vi "UHR-Fleezers Control (host) - 10.8.vi"() -> ()   [LabVIEW 2013] (continued)
            n1214 = xnode "Read/Write Control"("FPGA VI Reference In"=w3569, "error in"=w3568, "AI to FIFO"=w3570, "APD to FIFO"=w3570, "Start scan"=w3570) -> ("FPGA VI Reference Out"=w3567:T19, "error out"=w3566:errorcluster)
          }
          frame True {
            w3594 = FALSE ("1D or 2D Scan?")
            w3599 = TRUE ("AI to FIFO")
            # "Count for MCL loop"
            # "N total cycles"
            # "N steps"
            # "V_int"
            n1215 = local read "Scan Range (nm)"() -> (w3576:dbl)
            n1216 = local read "Number of F/B Scans (AOD)"() -> (w3593:u16)
            n1217 = Sign(1:w3576) -> (0:w3575:dbl)
            n1218 = Compound Arithmetic op=MULTIPLY(w3576, "MCL Step Position Ratio", "MCL/AOM Scale Tweak") -> (w3580:dbl)
            n1219 = Negate(x=w3575) -> (-x=w3572:dbl)
            n1220 = Multiply(x=w3572, y="MCL Step Increment (V_int)") -> (x*y=w3574:dbl)
            n1221 = Divide(x=w3580, y="MCL X Cal (nm/V)") -> (x/y=w3586:dbl)
            n1222 = Multiply(x=32767.0 ("y"), y=w3586) -> (x*y=w3592:dbl)
            n1223 = local read "Total Counts (ticks)"() -> (w3577:u32)
            n1224 = local read "Cycles/step (AOD)"() -> (w3588:u64)
            n1225 = local read "Scan steps (AOD)"() -> (w3589:u64)
            n1226 = Divide(x=w3592, y=10.0) -> (x/y=w3585:dbl)
            n1227 = Divide(x=w3585, y="MCL Step Increment (V_int)") -> (x/y=w3583:dbl)
            n1228 = Absolute Value(x=w3583) -> (abs(x)=w3571:dbl)
            n1229 = Compound Arithmetic op=MULTIPLY(w3589, w3588, w3577) -> (w3584:u64)
            n1230 = local write "wait to reset values"(w3599) -> ()
            n1231 = local write "MCL Scanning"(w3599) -> ()
            n1232 = Divide(x=w3584, y=w3571) -> (x/y=w3581:dbl)
            "MCL Count" <- w3581
            n1233 = xnode "Read/Write Control"("FPGA VI Reference In"=w3598, "error in"=w3597, "Scan steps (MCL)"=w3571, "Number of scans (MCL)"=w3593, "Cycles per step (MCL)"=u64 1, "Scan freq.  increment (MCL)"=w3574, "1D or 2D Scan?"=w3594, "MCL Scan Axis"=w3594, "Cont. Scan (MCL)"=w3594, "MCL count"=w3581) -> ("FPGA VI Reference Out"=w3596:T19, "error out"=w3595:errorcluster)
            n1234 = xnode "Read/Write Control"("FPGA VI Reference In"=w3596, "error in"=w3595, "AI to FIFO"=w3599, "APD to FIFO"=w3599, "Start scan"=w3599, "Start scan (MCL)"=w3599) -> ("FPGA VI Reference Out"=w3601:T19, "error out"=w3600:errorcluster)
          }
        }
        "Raster Scanning..." <- TRUE ("Scanning...")
      }
    }
    n1235 = And(x="Save scans", y=w2105) -> (x .and. y?=w2151:bool)
    n1236 = Compound Arithmetic op=OR("Start MCL Scan", "Confocal Image", "Confocal Linescan") -> (w2103:bool)
    n1237 = And(x="Save Data (MCL)", y=w2103) -> (x .and. y?=w2150:bool)
    n1238 = case "Start MCL raster scan" shown="True" w2103 {
      tunnel: w2153 -> [w3032 w3047]
      tunnel: w2152 -> [w3031 w3046]
      tunnel: [w3032 w3042] -> w1910
      tunnel: [w3031 w3041] -> w1909
      tunnel: [FALSE w3040] -> w2136
      tunnel: "Start MCL Scan" -> [_ w3035]
      tunnel: "Confocal Image" -> [_ w3034]
      tunnel: "Confocal Linescan" -> [_ _]
      frame False {
      }
      frame True {
        w3040 = TRUE
        n1239 = case shown="True" "Restart DMA? (MCL)" {
          tunnel: [w3092 w3094] -> w3045
          tunnel: [w3091 w3093] -> w3044
          tunnel: w3047 -> [w3092 w3097]
          tunnel: w3046 -> [w3091 w3096]
          frame False {
          }
          frame True {
            n1240 = call "reset FPGA DMA.vi"("error in"=w3096, "FPGA VI Reference In"=w3097) -> ("error out"=w3093:errorcluster, "FPGA VI Reference Out"=w3094:T19)
            n1241 = local write "Overflow (data lost)"(FALSE ("Overflow (data lost)")) -> ()
          }
        }
        n1242 = case shown="False" w3035 {
          selector: w3035 -> [_ w3051]
          tunnel: w3034 -> [w3050 _]
          tunnel: [w3050 w3051] -> w3033
          frame False {
            n1243 = property on="2D or 1D Scan" class="Bool (strict)"("Val(Sgnl)"=w3050) -> ()  [unwired: 2 in, 2 out]
            n1244 = property on="Confocal Image" class="Bool (strict)"("Value"=FALSE ("Start Confocal Map")) -> ()  [unwired: 2 in, 2 out]
          }
          frame True {
          }
        }
        n1245 = local write "MCL Scanning"(w3040) -> ()
        n1246 = local read "AO1"() -> (w3037:dbl)
        n1247 = local read "AO2"() -> (w3036:dbl)
        n1248 = case shown="True" "Center Scan" {
          tunnel: w3045 -> [w3058 w3090]
          tunnel: w3044 -> [w3057 w3089]
          tunnel: [w3056 w3088] -> w3042
          tunnel: [w3055 w3087] -> w3041
          tunnel: [w3053 w3074] -> w3039
          tunnel: [w3052 w3073] -> w3038
          tunnel: w3037 -> [w3053 w3079]
          tunnel: w3036 -> [w3052 w3082]
          tunnel: w3033 -> [_ _]
          frame False {
            w3054 = TRUE ("AI to FIFO")
            n1249 = xnode "Read/Write Control"("FPGA VI Reference In"=w3058, "error in"=w3057, "AI to FIFO"=w3054, "APD to FIFO"=w3054, "Start scan (MCL)"=w3054) -> ("FPGA VI Reference Out"=w3056:T19, "error out"=w3055:errorcluster)
          }
          frame True {
            w3086 = TRUE ("AI to FIFO")
            n1250 = local read "Scan steps (MCL)"() -> (w3065:u64)
            n1251 = local read "Scan lines (y)"() -> (w3061:u64)
            n1252 = local read "Fast Scan Dir"() -> (w3072:bool)
            n1253 = local read "Actual MCL Inc (V)"() -> (w3062:dbl)
            n1254 = Decrement(x=w3061) -> (x-1=w3060:u64)
            n1255 = Decrement(x=w3065) -> (x-1=w3064:u64)
            n1256 = Multiply(x=w3062, y=w3060) -> (x*y=w3059:dbl)
            n1257 = Divide(x=w3059, y=2.0) -> (x/y=w3069:dbl)
            n1258 = Multiply(x=w3062, y=w3064) -> (x*y=w3063:dbl)
            n1259 = Divide(x=w3063, y=2.0) -> (x/y=w3068:dbl)
            n1260 = Select(t=w3068, s=w3072, f=w3069) -> (s? t:f=w3067:dbl)
            n1261 = Select(t=w3069, s=w3072, f=w3068) -> (s? t:f=w3071:dbl)
            n1262 = Subtract(x=w3079, y=w3071) -> (x-y=w3070:dbl)
            n1263 = Subtract(x=w3082, y=w3067) -> (x-y=w3066:dbl)
            n1264 = local read "2D or 1D Scan"() -> (w3084:bool)
            n1265 = Not(x=w3072) -> (.not. x?=w3078:bool)
            n1266 = Not(x=w3084) -> (.not. x?=w3080:bool)
            n1267 = And(x=w3072, y=w3080) -> (x .and. y?=w3081:bool)
            n1268 = And(x=w3080, y=w3078) -> (x .and. y?=w3083:bool)
            n1269 = Select(t=w3082, s=w3083, f=w3066) -> (s? t:f=w3073:dbl)
            n1270 = Select(t=w3079, s=w3081, f=w3070) -> (s? t:f=w3074:dbl)
            n1271 = call "Volt to I16.vi"("Voltage In"=w3074) -> ("I16 Voltage Out"=w3077:i16)
            n1272 = call "Volt to I16.vi"("Voltage In"=w3073) -> ("I16 Voltage Out"=w3076:i16)
            n1273 = xnode "Read/Write Control"("FPGA VI Reference In"=w3090, "error in"=w3089, "AI to FIFO"=w3086, "APD to FIFO"=w3086, "Start scan (MCL)"=w3086, "AO1"=w3077, "AO2"=w3076) -> ("FPGA VI Reference Out"=w3088:T19, "error out"=w3087:errorcluster)
          }
        }
        "Initial Y" <- w3039
        "Initial X" <- w3038
        "wait to reset values" <- w3040
      }
    }
    n1274 = local read "Trap Pos Elements/DMA read"() -> (w1984:u32)
    n1275 = local read "Trap AI Elements/DMA read"() -> (w1908:u32)
    n1276 = local read "APD Elements/DMA read"() -> (w2027:u32)
    n1277 = local read "Trap AI FIFO Depth"() -> (w2200:u32)
    n1278 = xnode "Invoke Method"("FPGA VI Reference In"=w1910, "error in"=w1909, "Number of Elements"=w1984, "Timeout (ms)"=-1) -> ("Data"=w1948:u16[], "Elements Remaining"=→"Trap Pos FIFO El Remaining":u32)  [unwired: 2 out]
    n1279 = xnode "Invoke Method"("FPGA VI Reference In"=w1910, "error in"=w1909, "Number of Elements"=w1908, "Timeout (ms)"=-1 ("Timeout")) -> ("FPGA VI Reference Out"=w1912:T19, "error out"=w1911:errorcluster, "Data"=w1907:i16[], "Elements Remaining"=w1913:u32)
    "Trap AI FIFO El. Rem." <- w1913
    n1280 = xnode "Get APD Data"("FPGA VI Reference In"=w1910, "error in"=w1909, "Number of Elements"=w2027, "Timeout (ms)"=-1) -> ("Data"=w2026:u32[], "Elements Remaining"=→"APD FIFO Elements Remaining":u32)  [unwired: 2 out]
    n1281 = Subtract(x=w2200, y=w1908) -> (x-y=w2199:u32)
    n1282 = Decimate 1D Array(w1948) -> (w1945:u16[], w1947:u16[], w1946:u16[])
    n1283 = Divide(x=w1913, y=w2199) -> (x/y=w2198:dbl)
    "Buffer Status" <- w2198
    n1284 = To Unsigned Long Integer(number=w1945) -> (unsigned 32bit integer=w1944:u32[])
    n1285 = Join Numbers(hi=w1947, lo=w1946) -> ((hi.lo)=w1943:u32[])
    n1286 = Equal?(x=w2198, y=1.0) -> (x = y?=w2196:bool)
    n1287 = Join Numbers(hi=w1944, lo=w1943) -> ((hi.lo)=w1937:u64[])
    n1288 = call "IR AOM word to freq - vec.vi"("Frequency Word In (double vec)"=w1937) -> ("Frequency Out"=w1983:dbl[])
    n1289 = case "Alert buffer overflow" shown="True" w2196 {
      frame False {
      }
      frame True {
        n1290 = call <vilib>:"Beep.vi"() -> ()  [unwired: 3 in, 9 out]
        "Overflow (data lost)" <- TRUE ("Overflow (data lost)")
      }
    }
    n1291 = Decimate 1D Array(w1983) -> (w1982:dbl[], w1981:dbl[])
    n1292 = Array Size(array=w1907) -> (size(s)=→"Waveform Chart":i32)
    n1293 = Build Array(w1982, w1981) -> (w1980:dbl[][])
    n1294 = local read "Trap Sets"() -> (w2064:u32)
    n1295 = case "Deinterlace trap data, average down PSD" shown="2" w2064 {
      tunnel: w1907 -> [w3127 w3192]
      tunnel: [w3124 w3189] -> w2057
      tunnel: [w3127 w3191] -> w1940
      tunnel: "Detector Type" -> [w3126 w3187]
      tunnel: [w3125 w3190] -> w2056
      tunnel: [w3123 w3188] -> w2171
      frame 1, Default {
        n1296 = Divide(x=w3127, y=3276.7) -> (x/y=w3128:dbl[])
        n1297 = Decimate 1D Array(w3128) -> (w3137:dbl[], w3136:dbl[], w3135:dbl[], w3134:dbl[], w3133:dbl[], w3132:dbl[], w3131:dbl[], w3130:dbl[])
        n1298 = case shown="\"IR-QPD + PSD + FB-QPD position\"" w3126 {
          tunnel: w3137 -> [w3161 w3186]
          tunnel: w3136 -> [w3160 w3185]
          tunnel: w3135 -> [w3145 w3163]
          tunnel: w3134 -> [w3146 w3173]
          tunnel: w3133 -> [w3159 w3184]
          tunnel: w3132 -> [w3158 w3183]
          tunnel: w3131 -> [w3142 w3164]
          tunnel: w3130 -> [w3141 w3162]
          tunnel: [w3140 w3170] -> w3125
          tunnel: [w3139 w3169] -> w3124
          tunnel: [w3138 w3168] -> w3123
          frame "IR-QPD + PSD + FB-QPD", Default {
            w3138 = 0  # Channel pattern
            n1299 = Divide(x=w3161, y=w3146) -> (x/y=w3148:dbl[])
            n1300 = Divide(x=w3160, y=w3146) -> (x/y=w3147:dbl[])
            n1301 = Divide(x=w3159, y=w3142) -> (x/y=w3144:dbl[])
            n1302 = Divide(x=w3158, y=w3141) -> (x/y=w3143:dbl[])
            n1303 = Build Array(w3148, w3147, w3146, w3145, w3144, w3143, w3142, w3141) -> (w3139:dbl[][])
            n1304 = Bundle("T1 Y", "T1 X", "T1 Sum", "FB Sum", "PSD Y", "PSD X", "PSD Y Sum", "PSD X Sum") -> (w3157:T45)  [unwired: 1 out]
            n1305 = Cluster To Array(cluster=w3157) -> (array=w3140:string[])
          }
          frame "IR-QPD + PSD + FB-QPD position" {
            w3168 = 3  # Channel pattern
            n1306 = Negate(x=w3164) -> (-x=w3165:dbl[])
            n1307 = Divide(x=w3186, y=w3173) -> (x/y=w3175:dbl[])
            n1308 = Divide(x=w3185, y=w3173) -> (x/y=w3174:dbl[])
            n1309 = Divide(x=w3184, y=w3164) -> (x/y=w3172:dbl[])
            n1310 = Divide(x=w3183, y=w3165) -> (x/y=w3171:dbl[])
            n1311 = Build Array(w3175, w3174, w3173, w3162, w3163, w3172, w3171, w3164) -> (w3169:dbl[][])
            n1312 = Bundle("T1 Y", "T1 X", "T1 Sum", "FB X", "FB Sum", "PSD Y", "PSD X", "PSD Y Sum") -> (w3182:T45)  [unwired: 1 out]
            n1313 = Cluster To Array(cluster=w3182) -> (array=w3170:string[])
          }
        }
      }
      frame 2 {
        n1314 = case shown="\"UCB Fleezers 052511\"" w3187 {
          tunnel: w3192 -> [w3254 w3321 w3349 w3456]
          tunnel: [w3193 w3313 w3344 w3387] -> w3191
          tunnel: [w3220 w3304 w3346 w3434] -> w3190
          tunnel: [w3219 w3268 w3323 w3401] -> w3189
          tunnel: [w3213 w3303 w3386 w3432] -> w3188
          frame "IR-QPD + PSD + FB-QPD", Default {
            w3213 = 1  # Channel pattern
            # "time average x2 the 4th signal and the 4 psd signals (detection laser)"
            # "deinterlace 3 signals from qpd"
            n1315 = Decimate 1D Array(w3254) -> (w3253:i16[], w3252:i16[], w3218:i16[], w3251:i16[], w3241:i16[], w3239:i16[], w3238:i16[], w3236:i16[])
            n1316 = call "downsample 1D array - double.vi"("Ave N"=2.0, "Array In"=w3241) -> ("Array Out"=w3240:dbl[])  [unwired: 1 out]
            n1317 = call "downsample 1D array - double.vi"("Ave N"=2.0, "Array In"=w3236) -> ("Array Out"=w3235:dbl[])  [unwired: 1 out]
            n1318 = call "downsample 1D array - double.vi"("Ave N"=2.0, "Array In"=w3238) -> ("Array Out"=w3237:dbl[])  [unwired: 1 out]
            n1319 = call "downsample 1D array - double.vi"("Ave N"=2.0, "Array In"=w3239) -> ("Array Out"=w3221:dbl[])  [unwired: 1 out]
            n1320 = Decimate 1D Array(w3253) -> (w3250:i16[], w3222:i16[])
            n1321 = Decimate 1D Array(w3252) -> (w3249:i16[], w3247:i16[])
            n1322 = Decimate 1D Array(w3251) -> (w3248:i16[], w3246:i16[])
            n1323 = Decimate 1D Array(w3218) -> (w3217:i16[], w3216:i16[])
            n1324 = Interleave 1D Arrays(w3250, w3249, w3248, w3222, w3247, w3246, w3217, w3216, w3240, w3221, w3237, w3235) -> (w3234:dbl[])
            n1325 = To Word Integer(number=w3234) -> (16bit integer=w3193:i16[])
            n1326 = Divide(x=w3234, y=3276.7) -> (x/y=w3233:dbl[])
            n1327 = Decimate 1D Array(w3233) -> (w3232:dbl[], w3231:dbl[], w3230:dbl[], w3229:dbl[], w3228:dbl[], w3227:dbl[], w3215:dbl[], w3214:dbl[], w3226:dbl[], w3225:dbl[], w3224:dbl[], w3223:dbl[])
            n1328 = Divide(x=w3232, y=w3230) -> (x/y=w3200:dbl[])
            n1329 = Divide(x=w3231, y=w3230) -> (x/y=w3199:dbl[])
            n1330 = Divide(x=w3229, y=w3227) -> (x/y=w3198:dbl[])
            n1331 = Divide(x=w3228, y=w3227) -> (x/y=w3197:dbl[])
            n1332 = Divide(x=w3226, y=w3224) -> (x/y=w3196:dbl[])
            n1333 = Divide(x=w3225, y=w3223) -> (x/y=w3195:dbl[])
            n1334 = Bundle("T1 Y", "T1 X", "T1 Sum", "T2 Y", "T2 X", "T2 Sum", "T1 FB Sum", "T2 FB Sum", "PSD Y", "PSD X", "PSD Y Sum", "PSD X Sum") -> (w3201:T46)  [unwired: 1 out]
            n1335 = Build Array(w3200, w3199, w3230, w3198, w3197, w3227, w3215, w3214, w3196, w3195, w3224, w3223) -> (w3219:dbl[][])
            n1336 = Cluster To Array(cluster=w3201) -> (array=w3220:string[])
          }
          frame "IR-QPD + PSD + FB-QPD X position" {
            w3303 = 2  # Channel pattern
            # "convert\nADC numbers\nto volts"
            # "time average x2 the 3 psd signals (detection laser)"
            # "deinterlace 3 signals from qpds"
            n1337 = Decimate 1D Array(w3321) -> (w3320:i16[], w3319:i16[], w3256:i16[], w3257:i16[], w3266:i16[], w3263:i16[], w3260:i16[], w3291:i16[])
            n1338 = Decimate 1D Array(w3320) -> (w3318:i16[], w3305:i16[])
            n1339 = call "downsample 1D array - I16.vi"("Ave N"=2.0, "Array In"=w3266) -> ("Array Out"=w3264:i16[])  [unwired: 1 in]
            n1340 = call "downsample 1D array - I16.vi"("Ave N"=2.0, "Array In"=w3263) -> ("Array Out"=w3261:i16[])  [unwired: 1 in]
            n1341 = Decimate 1D Array(w3319) -> (w3317:i16[], w3315:i16[])
            n1342 = Decimate 1D Array(w3257) -> (w3316:i16[], w3314:i16[])
            n1343 = Decimate 1D Array(w3291) -> (w3290:i16[], w3288:i16[])
            n1344 = Decimate 1D Array(w3256) -> (w3289:i16[], w3287:i16[])
            n1345 = call "downsample 1D array - I16.vi"("Ave N"=2.0, "Array In"=w3260) -> ("Array Out"=w3258:i16[])  [unwired: 1 in]
            n1346 = Interleave 1D Arrays(w3318, w3317, w3316, w3305, w3315, w3314, w3290, w3289, w3288, w3287, w3264, w3261, w3258) -> (w3313:i16[])
            n1347 = Divide(x=w3313, y=3276.7) -> (x/y=w3312:dbl[])
            n1348 = Decimate 1D Array(w3312) -> (w3311:dbl[], w3310:dbl[], w3309:dbl[], w3308:dbl[], w3307:dbl[], w3306:dbl[], w3279:dbl[], w3277:dbl[], w3276:dbl[], w3274:dbl[], w3273:dbl[], w3272:dbl[], w3269:dbl[])
            n1349 = Divide(x=w3311, y=w3309) -> (x/y=w3295:dbl[])
            n1350 = Divide(x=w3310, y=w3309) -> (x/y=w3294:dbl[])
            n1351 = Divide(x=w3308, y=w3306) -> (x/y=w3293:dbl[])
            n1352 = Divide(x=w3307, y=w3306) -> (x/y=w3292:dbl[])
            n1353 = Divide(x=w3279, y=w3277) -> (x/y=w3278:dbl[])
            n1354 = Divide(x=w3276, y=w3274) -> (x/y=w3275:dbl[])
            n1355 = Divide(x=w3273, y=w3269) -> (x/y=w3271:dbl[])
            n1356 = Negate(x=w3269) -> (-x=w3267:dbl[])
            n1357 = Divide(x=w3272, y=w3267) -> (x/y=w3270:dbl[])
            n1358 = Bundle("T1 Y", "T1 X", "T1 Sum", "T2 Y", "T2 X", "T2 Sum", "T1 FB X", "T1 FB Sum", "T2 FB X", "T2 FB Sum", "PSD Y", "PSD X", "PSD Y Sum") -> (w3296:T47)  [unwired: 1 out]
            n1359 = Build Array(w3295, w3294, w3309, w3293, w3292, w3306, w3278, w3277, w3275, w3274, w3271, w3270, w3269) -> (w3268:dbl[][])
            n1360 = Cluster To Array(cluster=w3296) -> (array=w3304:string[])
          }
          frame "UCB Fleezers 052511" {
            w3386 = 2  # Channel pattern
            n1361 = Decimate 1D Array(w3349) -> (w3384:i16[], w3383:i16[], w3348:i16[], w3347:i16[], w3341:i16[], w3338:i16[], w3337:i16[], w3336:i16[])
            n1362 = Decimate 1D Array(w3384) -> (w3382:i16[], w3367:i16[])
            n1363 = Decimate 1D Array(w3383) -> (w3381:i16[], w3379:i16[])
            n1364 = Decimate 1D Array(w3348) -> (w3380:i16[], w3378:i16[])
            n1365 = Decimate 1D Array(w3347) -> (w3343:i16[], w3342:i16[])
            n1366 = Decimate 1D Array(w3341) -> (w3340:i16[], w3339:i16[])
            n1367 = call "downsample 1D array - I16.vi"("Ave N"=2.0, "Array In"=w3338) -> ("Array Out"=w3335:i16[])  [unwired: 1 in]
            n1368 = call "downsample 1D array - I16.vi"("Ave N"=2.0, "Array In"=w3337) -> ("Array Out"=w3334:i16[])  [unwired: 1 in]
            n1369 = call "downsample 1D array - I16.vi"("Ave N"=2.0, "Array In"=w3336) -> ("Array Out"=w3333:i16[])  [unwired: 1 in]
            n1370 = Interleave 1D Arrays(w3382, w3381, w3380, w3367, w3379, w3378, w3343, w3340, w3342, w3339, w3335, w3334, w3333) -> (w3344:i16[])
            n1371 = Divide(x=w3344, y=3276.7) -> (x/y=w3374:dbl[])
            n1372 = Decimate 1D Array(w3374) -> (w3373:dbl[], w3372:dbl[], w3371:dbl[], w3370:dbl[], w3369:dbl[], w3368:dbl[], w3332:dbl[], w3330:dbl[], w3329:dbl[], w3327:dbl[], w3326:dbl[], w3325:dbl[], w3324:dbl[])
            n1373 = Divide(x=w3373, y=w3371) -> (x/y=w3354:dbl[])
            n1374 = Divide(x=w3372, y=w3371) -> (x/y=w3353:dbl[])
            n1375 = Divide(x=w3370, y=w3368) -> (x/y=w3352:dbl[])
            n1376 = Divide(x=w3369, y=w3368) -> (x/y=w3351:dbl[])
            n1377 = Divide(x=w3332, y=w3330) -> (x/y=w3331:dbl[])
            n1378 = Divide(x=w3329, y=w3327) -> (x/y=w3328:dbl[])
            n1379 = Bundle("T1 Y", "T1 X", "T1 Sum", "T2 Y", "T2 X", "T2 Sum", "T1 FB X", "T2 FB Sum", "T2 FB X", "T2 FB Sum", "PSD Y", "PSD X", "PSD Sum") -> (w3355:T47)  [unwired: 1 out]
            n1380 = Build Array(w3354, w3353, w3371, w3352, w3351, w3368, w3331, w3330, w3328, w3327, w3326, w3325, w3324) -> (w3323:dbl[][])
            n1381 = Cluster To Array(cluster=w3355) -> (array=w3346:string[])
          }
          frame "IR-QPD + PSD + FB-QPD XY positions" {
            w3432 = 4  # Channel pattern
            # "time average x2 the 3 psd signals (detection laser)"
            # "deinterlace 3 signals from qpds"
            n1382 = Decimate 1D Array(w3456) -> (w3455:i16[], w3454:i16[], w3433:i16[], w3453:i16[], w3399:i16[], w3445:i16[], w3444:i16[], w3421:i16[])
            n1383 = Decimate 1D Array "QPD Y"(w3455) -> (w3452:i16[], w3435:i16[])
            n1384 = call "downsample 1D array - double.vi"("Ave N"=2.0, "Array In"=w3445) -> ("Array Out"=w3420:dbl[])  [unwired: 1 out]
            n1385 = call "downsample 1D array - double.vi"("Ave N"=2.0, "Array In"=w3444) -> ("Array Out"=w3419:dbl[])  [unwired: 1 out]
            n1386 = Decimate 1D Array "Feedback Sum"(w3433) -> (w3417:i16[], w3415:i16[])
            n1387 = Decimate 1D Array "Feedback Y"(w3399) -> (w3398:i16[], w3397:i16[])
            n1388 = Decimate 1D Array "Feedback X"(w3421) -> (w3418:i16[], w3416:i16[])
            n1389 = Decimate 1D Array "QPD Sum"(w3453) -> (w3450:i16[], w3448:i16[])
            n1390 = Decimate 1D Array "QPD X"(w3454) -> (w3451:i16[], w3449:i16[])
            n1391 = Interleave 1D Arrays(w3452, w3451, w3450, w3435, w3449, w3448, w3398, w3418, w3417, w3397, w3416, w3415, w3420, w3419) -> (w3443:dbl[])
            n1392 = To Word Integer(number=w3443) -> (16bit integer=w3387:i16[])
            n1393 = Divide(x=w3443, y=3276.7) -> (x/y=w3442:dbl[])
            n1394 = Decimate 1D Array(w3442) -> (w3441:dbl[], w3440:dbl[], w3439:dbl[], w3438:dbl[], w3437:dbl[], w3436:dbl[], w3394:dbl[], w3408:dbl[], w3392:dbl[], w3393:dbl[], w3406:dbl[], w3390:dbl[], w3404:dbl[], w3402:dbl[])
            n1395 = Divide(x=w3441, y=w3439) -> (x/y=w3425:dbl[])
            n1396 = Divide(x=w3440, y=w3439) -> (x/y=w3424:dbl[])
            n1397 = Divide(x=w3438, y=w3436) -> (x/y=w3423:dbl[])
            n1398 = Divide(x=w3437, y=w3436) -> (x/y=w3422:dbl[])
            n1399 = Divide(x=w3394, y=w3392) -> (x/y=w3391:dbl[])
            n1400 = Divide(x=w3408, y=w3392) -> (x/y=w3407:dbl[])
            n1401 = Divide(x=w3393, y=w3390) -> (x/y=w3389:dbl[])
            n1402 = Divide(x=w3406, y=w3390) -> (x/y=w3405:dbl[])
            n1403 = Negate(x=w3402) -> (-x=w3400:dbl[])
            n1404 = Divide(x=w3404, y=w3400) -> (x/y=w3403:dbl[])
            n1405 = Bundle("T1 Y", "T1 X", "T1 Sum", "T2 Y", "T2 X", "T2 Sum", "T1 FB Y", "T1 FB X", "T1 FB Sum", "T2 FB Y", "T2 FB X", "T2 FB Sum", "PSD X", "PSD Y Sum") -> (w3388:T48)  [unwired: 1 out]
            n1406 = Build Array(w3425, w3424, w3439, w3423, w3422, w3436, w3391, w3407, w3392, w3389, w3405, w3390, w3403, w3402) -> (w3401:dbl[][])
            n1407 = Cluster To Array(cluster=w3388) -> (array=w3434:string[])
          }
        }
      }
    }
    "AI labels" <- w2056
    n1408 = Decimate 1D Array(w2026) -> (w2054:u32[], w1990:u32[])
    n1409 = local read "DMA Update Period (s)"() -> (w2065:dbl)
    n1410 = local read "BD 1 Frequency 2 (MHz)"() -> (w1932:dbl)
    n1411 = local read "BD 1 Frequency 1 (MHz)"() -> (w1933:dbl)
    n1412 = Build Array(w2054, w1990) -> (w2133:u32[][])
    n1413 = local read "Data Period (s)"() -> (w2039:dbl)
    n1414 = Decimate 1D Array(w1940) -> (w1963:i16[], w1962:i16[], w1960:i16[], w1959:i16[])  [unwired: 9 out]
    n1415 = To Double Precision Float(number=w2133) -> (double precision float=w2134:dbl[][])
    n1416 = local read "APD Integration Time (s)"() -> (w2003:dbl)
    n1417 = Divide(x=w1963, y=w1962) -> (x/y=w1964:dbl[])
    n1418 = Divide(x=w1960, y=w1959) -> (x/y=w1961:dbl[])
    n1419 = feedback #1(0.0) -> (w1977:dbl)
    n1420 = Add(x=w2065, y=w1977) -> (x+y=w2173:dbl)
    n1421 = feedback-in #1(w2173) -> ()
    n1422 = local read "AOM X Cal (nm/MHz)"() -> (w1930:dbl)
    n1423 = To Time Stamp(1:w1977) -> (0:w1976:timestamp)
    n1424 = Split 1D Array(array=w1964, index="N El. to Ave.") -> (second subarray=w1967:dbl[])  [unwired: 1 out]
    n1425 = Split 1D Array(array=w1961, index="N El. to Ave.") -> (second subarray=w1966:dbl[])  [unwired: 1 out]
    n1426 = local read "Trap X AI1 (DMA)"() -> (w1965:T13)
    n1427 = Multiply(x=w2039, y="Trap Disp. Downsample") -> (x*y=w1978:dbl)
    "Display Period (s)" <- w1978
    n1428 = Bundle("BD 1 Frequency 1 (MHz)"=w1933, "BD 1 Frequency 2 (MHz)"=w1932) -> (w1934:T49)  [unwired: 1 out]
    n1429 = for "Trap AI" {
      tunnel: [w3122] -> w2167 mode=indexing
      tunnel: w1976 -> [w3112]
      tunnel: "Trap Disp. Downsample" -> [w3120]
      tunnel: w2057 -> [w3118] mode=indexing
      tunnel: w2039 -> [w3117]
      tunnel: w2056 -> [w3116] mode=indexing
      tunnel: w1975 -> [w3115]
      tunnel: [w3114] -> w2014 mode=indexing
      tunnel: w1978 -> [w3113]
      n1430 = Bundle By Name("Y"=w3118, "dt"=w3117) -> (w3119:waveform(dbl))  [unwired: 1 out]
      n1431 = Set Waveform Attribute(5:w3116, 6:w3115, 7:w3119) -> (3:w3114:waveform(dbl))  [unwired: 1 in, 2 out]
      n1432 = call "downsample 1D array - double.vi"("Ave N"=w3120, "Array In"=w3118) -> ("Array Out"=w3121:dbl[])  [unwired: 1 out]
      n1433 = Bundle By Name(cluster=w3114, "t0"=w3112, "Y"=w3121, "dt"=w3113) -> (w3122:waveform(dbl))
    }
    n1434 = call-poly <vilib>:"Mean.vi"("X"=w1966) -> ("mean"=w1954:dbl)  [unwired: 1 out]
    n1435 = call-poly <vilib>:"Mean.vi"("X"=w1967) -> ("mean"=w1955:dbl)  [unwired: 1 out]
    n1436 = Cluster To Array(cluster=w1934) -> (array=w1931:dbl[])
    n1437 = Reciprocal(x=w1978) -> (1/x=→"Trap Disp. Freq. (Hz)":dbl)
    n1438 = local read "Data points/scans (MCL)"() -> (w2145:dbl)
    n1439 = To Fixed-Point(number=w1954) -> (fixed-point=w1952:fxp<+/-,16,1>)  [unwired: 1 in]
    n1440 = To Fixed-Point(number=w1955) -> (fixed-point=w1953:fxp<+/-,16,1>)  [unwired: 1 in]
    n1441 = Bundle("Trap 1 Pos.", "Trap 2 Pos.") -> (w1974:cluster{string, string})  [unwired: 1 out]
    n1442 = Bundle By Name(cluster=w1965, "Set 1"=w1953, "Set 2"=w1952) -> (→"Trap X AI1 (DMA)":T13)
    n1443 = Cluster To Array(cluster=w1974) -> (array=w1971:string[])
    n1444 = for "Trap Position" {
      tunnel: w1980 -> [w2371] mode=indexing
      tunnel: "Trap Disp. Downsample" -> [w2370]
      tunnel: w1978 -> [w2368]
      tunnel: w1976 -> [w2367]
      tunnel: w1975 -> [w2365]
      tunnel: w1971 -> [w2364] mode=indexing
      tunnel: [w2363] -> w1929 mode=indexing
      tunnel: w1931 -> [w2361] mode=indexing
      tunnel: w1930 -> [w2359]
      n1445 = call "downsample 1D array - double.vi"("Ave N"=w2370, "Array In"=w2371) -> ("Array Out"=w2369:dbl[])  [unwired: 1 out]
      n1446 = Subtract(x=w2369, y=w2361) -> (x-y=w2362:dbl[])
      n1447 = Multiply(x=w2359, y=w2362) -> (x*y=w2360:dbl[])
      n1448 = Bundle By Name("Y"=w2360, "dt"=w2368, "t0"=w2367) -> (w2366:waveform(dbl))  [unwired: 1 out]
      n1449 = Set Waveform Attribute(5:w2364, 6:w2365, 7:w2366) -> (3:w2363:waveform(dbl))  [unwired: 1 in, 2 out]
    }
    "Trap Positions" <- w1929
    n1450 = Bundle("APD 1", "APD 2") -> (w2166:cluster{string, string})  [unwired: 1 out]
    n1451 = Cluster To Array(cluster=w2166) -> (array=w2163:string[])
    n1452 = for "APD" {
      tunnel: w2134 -> [w3101] mode=indexing
      tunnel: w2003 -> [w3109]
      tunnel: [w3105] -> w2010 mode=indexing
      tunnel: "APD Disp. Scale" -> [w3106]
      tunnel: w1975 -> [w3104]
      tunnel: w2163 -> [w3103] mode=indexing
      tunnel: "APD Disp. Downsample" -> [w3099]
      tunnel: [w3102] -> w2162
      tunnel: w1976 -> [w3098]
      n1453 = call "integrate 1D array interval - double.vi"("Ave N"=w3099, "Array In"=w3101) -> ("Array Out"=w3100:dbl[])  [unwired: 1 out]
      n1454 = Multiply(x=w3109, y=w3099) -> (x*y=w3102:dbl)
      n1455 = Divide(x=w3100, y=w3106) -> (x/y=w3107:dbl[])
      n1456 = Bundle By Name("t0"=w3098, "Y"=w3107, "dt"=w3102) -> (w3108:waveform(dbl))  [unwired: 1 out]
      n1457 = Set Waveform Attribute(5:w3103, 6:w3104, 7:w3108) -> (3:w3105:waveform(dbl))  [unwired: 1 in, 2 out]
    }
    "APD Display Period (s)" <- w2162
    n1458 = Reciprocal(x=w2162) -> (1/x=→"APD Display Freq. (Hz)":dbl)
    n1459 = local read "Display Period (s)"() -> (w2038:dbl)
    n1460 = Increment(x=w2145) -> (x+1=w2146:dbl)
    n1461 = Index Array(array=w1929, index=0) -> (element=w1927:waveform(dbl))
    n1462 = To Double Precision Float(number=w2054) -> (double precision float=w2053:dbl[])
    n1463 = feedback #2(w2146) -> (w2149:dbl)
    n1464 = Select(t=0, s=w2136, f=w2149) -> (s? t:f=w2142:dbl)
    n1465 = Array Size(array=w2053) -> (size(s)=w2148:i32)
    n1466 = Add(x=w2148, y=w2142) -> (x+y=w2143:dbl)
    n1467 = Unbundle By Name(w1927) -> ("Y"=w1925:dbl[])
    n1468 = feedback #3(w2054) -> (w2132:u32[])
    n1469 = Build Array (concatenate)(w2132, w2054) -> (w2129:u32[])
    n1470 = feedback #4(w1990) -> (w2009:u32[])
    n1471 = Divide(x="Bead Sep. Int. Time (s)", y=w2038) -> (x/y=w1923:dbl)
    n1472 = Build Array (concatenate)(w2009, w1990) -> (w2008:u32[])
    n1473 = Greater?(x=w2143, y=w2145) -> (0:w2144:bool)
    n1474 = feedback #5(w1925) -> (w1926:dbl[])
    n1475 = Build Array (concatenate)(w1925, w1926) -> (w1924:dbl[])
    n1476 = Select(t=w2142, s=w2144, f=w2143) -> (s? t:f=w2141:dbl)
    n1477 = feedback-in #2(w2141) -> ()
    n1478 = Array Size(array=w2129) -> (size(s)=w2126:i32)
    n1479 = Array Size(array=w2054) -> (size(s)=w2128:i32)
    n1480 = local read "MCL Scanning"() -> (w2139:bool)
    n1481 = local read "APD Integration Time (s)"() -> (w2017:dbl)
    n1482 = Build Array (concatenate)(w2010, w2167) -> (w2012:waveform(dbl)[])
    "All Signals" <- w2012
    n1483 = Split 1D Array(array=w1924, index=w1923) -> (first subarray=w1917:dbl[])  [unwired: 1 out]
    n1484 = feedback-in #5(w1917) -> ()
    n1485 = Multiply(x=w2128, y="APD Ave N") -> (x*y=w2127:dbl)
    n1486 = Greater?(x=w2126, y=w2127) -> (0:w2130:bool)
    n1487 = Not(x=w2144) -> (.not. x?=w2138:bool)
    n1488 = To Double Precision Float(number=w1990) -> (double precision float=w1989:dbl[])
    n1489 = call-poly <vilib>:"Mean.vi"("X"=w1917) -> ("mean"=w1916:dbl)  [unwired: 1 out]
    "Mean T1 Position (nm)" <- w1916
    n1490 = Subtract(x=w1917, y=w1916) -> (x-y=w1922:dbl[])
    n1491 = Square(x=w1922) -> (x^2=w1921:dbl[])
    n1492 = And(x=w2138, y=w2139) -> (x .and. y?=w2140:bool)
    n1493 = call-poly <vilib>:"Mean.vi"("X"=w1921) -> ("mean"=w1920:dbl)  [unwired: 1 out]
    n1494 = case shown="True" w2130 {
      tunnel: w2129 -> [w2882 w2889]
      tunnel: [w2882 w2887] -> w2070
      tunnel: w2127 -> [_ w2884]
      tunnel: w2126 -> [_ w2888]
      tunnel: w2008 -> [w2881 w2886]
      tunnel: [w2881 w2883] -> w2005
      frame False {
      }
      frame True {
        n1495 = Subtract(x=w2888, y=w2884) -> (x-y=w2885:dbl)
        n1496 = Array Subset(array=w2889, index=w2885, length=w2884) -> (w2887:u32[])
        n1497 = Array Subset(array=w2886, index=w2885, length=w2884) -> (w2883:u32[])
      }
    }
    n1498 = feedback-in #3(w2070) -> ()
    n1499 = feedback-in #4(w2005) -> ()
    n1500 = Or(x=w2140, y=w2136) -> (x .or. y?=w2137:bool)
    n1501 = Square Root(x=w1920) -> (sqrt(x)=w1919:dbl)
    n1502 = Equal?(x="Tab Control 6", y=T36."High Res Display") -> (x = y?=w2060:bool)
    n1503 = Multiply(x="APD Disp. Scale", y=w2010) -> (x*y=w2019:waveform(dbl)[])
    n1504 = Multiply(x="APD Disp. Downsample", y=w2017) -> (x*y=w2015:dbl)
    n1505 = Multiply(x=10.0, y=w1919) -> (x*y=→"Trap 1 Position RMS (A)":dbl)
    n1506 = Divide(x=w2019, y=w2015) -> (x/y=w1987:waveform(dbl)[])
    n1507 = Index Array(array=w1987, index=0) -> (element=w1997:waveform(dbl))
    n1508 = case "For computing FFTs for display" shown="True" "Compute FFT" {
      tunnel: w2014 -> [_ w3636]
      frame False {
      }
      frame True {
        n1509 = Build Array("FFT 1 Choice 1", "FFT 1 Choice 2", "FFT 2 Choice 1", "FFT 2 Choice 2") -> (w3629:u16[])
        n1510 = Array Size(array=w3636) -> (size(s)=w3635:i32)
        n1511 = feedback-in #6(w3629) -> ()
        n1512 = feedback #6(u16[] [100, 100, 100, 100]) -> (w3630:u16[])
        n1513 = feedback-in #7("# Spectra to Ave.") -> ()
        n1514 = feedback #7("# Spectra to Ave.") -> (w3627:dbl)
        n1515 = Not Equal?(x="# Spectra to Ave.", y=w3627) -> (x != y?=w3626:bool)
        n1516 = Not Equal?(x=w3629, y=w3630) -> (x != y?=w3628:bool)
        n1517 = feedback #8(1.0) -> (w3613:dbl)
        n1518 = Compound Arithmetic op=OR("Reset FFT", w3628, w3626) -> (w3611:bool)
        n1519 = Select(t=1.0, s=w3611, f=w3613) -> (s? t:f=w3615:dbl)
        n1520 = Greater?(x=w3615, y="# Spectra to Ave.") -> (0:w3634:bool)
        n1521 = Increment(x=w3615) -> (x+1=w3614:dbl)
        n1522 = feedback-in #8(w3614) -> ()
        n1523 = local read "DMA Update Period (s)"() -> (w3609:dbl)
        n1524 = Multiply(x="# Spectra to Ave.", y=w3609) -> (x*y=→"Ave. Time (s)":dbl)
        n1525 = Build Array(cluster{"f0":dbl, "df":dbl, "magnitude":dbl[]} {"f0"=0.0, "df"=0.0, "magnitude"=[]} ("PSD")) -> (w3618:cluster{"f0":dbl, "df":dbl, "magnitude":dbl[]}[])
        n1526 = Build Array(w3618, w3618, w3618, w3618) -> (w3620:T50)
        n1527 = feedback #9(w3620) -> (w3625:T50)
        n1528 = for {
          N: 4 -> [_]
          tunnel: w3629 -> [w3658] mode=indexing
          tunnel: w3636 -> [w3659]
          tunnel: w3635 -> [w3661]
          tunnel: w3611 -> [w3654]
          tunnel: w3634 -> [w3653]
          tunnel: "# Spectra to Ave." -> [w3652]
          tunnel: [w3651] -> w3624 mode=indexing
          tunnel: w3625 -> [w3656] mode=indexing
          tunnel: [w3655] -> w3612 mode=indexing
          tunnel: w3615 -> [w3650]
          n1529 = Less?(x=w3658, y=w3661) -> (x < y?=w3660:bool)
          n1530 = Index Array(array=w3659, index=w3658) -> (element=w3657:waveform(dbl))
          n1531 = case shown="True" w3660 {
            tunnel: w3657 -> [_ w3678]
            tunnel: w3656 -> [w3663 w3676]
            tunnel: [w3663 w3664] -> w3655
            tunnel: w3654 -> [_ w3675]
            tunnel: w3653 -> [_ w3668]
            tunnel: w3652 -> [_ w3667]
            tunnel: [cluster{"f0":dbl, "df":dbl, "magnitude":dbl[]} {"f0"=0.0, "df"=0.0, "magnitude"=[]} ("PSD") w3669] -> w3651
            tunnel: w3650 -> [_ w3666]
            frame False {
            }
            frame True {
              n1532 = call <vilib>:"Std Deviation and Variance.vi"("X"=w3678) -> ("mean"=w3679:dbl)  [unwired: 1 in, 2 out]
              n1533 = Subtract(x=w3678, y=w3679) -> (x-y=w3677:waveform(dbl))
              n1534 = xnode "Spectral Measurements"("Signals"=w3677) -> ("PSD"=w3671:cluster{"f0":dbl, "df":dbl, "magnitude":dbl[]})  [unwired: 1 in, 1 out]
              n1535 = case shown="False" w3675 {
                tunnel: w3676 -> [w3688 _]
                tunnel: [w3684 w3693] -> w3664
                tunnel: w3671 -> [w3687 w3694]
                tunnel: w3668 -> [w3686 _]
                frame False {
                  n1536 = Build Array (concatenate)(w3688, w3687) -> (w3685:cluster{"f0":dbl, "df":dbl, "magnitude":dbl[]}[])
                  n1537 = case shown="True" w3686 {
                    tunnel: w3685 -> [w3689 w3692]
                    tunnel: [w3689 w3690] -> w3684
                    frame False {
                    }
                    frame True {
                      n1538 = Delete From Array(array=w3692, index=0) -> (array with subset deleted=w3690:cluster{"f0":dbl, "df":dbl, "magnitude":dbl[]}[])  [unwired: 1 in, 1 out]
                    }
                  }
                }
                frame True {
                  n1539 = Build Array(w3694) -> (w3693:cluster{"f0":dbl, "df":dbl, "magnitude":dbl[]}[])
                }
              }
              n1540 = for {
                tunnel: w3664 -> [w3683] mode=indexing
                tunnel: [w3682] -> w3674 mode=indexing
                workers-P: _ -> [_]
                n1541 = Unbundle By Name(w3683) -> ("magnitude"=w3682:dbl[])
              }
              n1542 = Transpose 2D Array(2D array=w3674) -> (transposed array=w3673:dbl[][])
              n1543 = for {
                tunnel: w3673 -> [w3681] mode=indexing
                tunnel: [w3680] -> w3672 mode=indexing
                workers-P: _ -> [_]
                n1544 = Add Array Elements(numeric array=w3681) -> (sum=w3680:dbl)
              }
              n1545 = Select(t=w3667, s=w3668, f=w3666) -> (s? t:f=w3665:dbl)
              n1546 = Divide(x=w3672, y=w3665) -> (x/y=w3670:dbl[])
              n1547 = Bundle By Name(cluster=w3671, "magnitude"=w3670) -> (w3669:cluster{"f0":dbl, "df":dbl, "magnitude":dbl[]})
            }
          }
        }
        n1548 = case shown="True" w3611 {
          tunnel: w3612 -> [w3643 w3649]
          tunnel: [w3643 w3644] -> w3610
          frame False {
          }
          frame True {
            n1549 = Array Subset(array=w3649, index (row)=0 ("index"), length (row)=4 ("length"), index (col)=0 ("index"), length (col)=1 ("length")) -> (w3644:T50)
          }
        }
        n1550 = feedback-in #9(w3610) -> ()
        n1551 = Split 1D Array(array=w3624, index=2) -> (first subarray=→"FFT 1":cluster{"f0":dbl, "df":dbl, "magnitude":dbl[]}[], second subarray=→"FFT 2":cluster{"f0":dbl, "df":dbl, "magnitude":dbl[]}[])
      }
    }
    n1552 = Index Array(array=w1987, index=1) -> (element=w1995:waveform(dbl))
    n1553 = case "For displaying the high resolution display (no downsampling)" shown="True" w2060 {
      tunnel: w2014 -> [_ w2391]
      frame False {
      }
      frame True {
        n1554 = Index Array(array=w2391, index="High Res. Display") -> (element=w2392:waveform(dbl))
        n1555 = call <vilib>:"Std Deviation and Variance.vi"("X"=w2392) -> ("mean"=w2399:dbl, "standard deviation"=w2404:dbl)  [unwired: 1 in, 1 out]
        "Mean Intensity" <- w2399
        "Sigma" <- w2404
        n1556 = Subtract(x=w2392, y=w2399) -> (x-y=w2398:waveform(dbl))
        n1557 = Select(t=w2398, s="Subtract mean", f=w2392) -> (s? t:f=→"1 Channel":waveform(dbl))
        n1558 = Divide(x=w2404, y=w2399) -> (x/y=→"Sigma/Mean":dbl)
        n1559 = feedback #10(1) -> (w2393:i32)
        n1560 = Greater Or Equal?(x=w2393, y="Slow mean N ave.") -> (x >= y?=w2406:bool)
        n1561 = Increment(x=w2393) -> (x+1=w2408:i32)
        n1562 = Select(t=1, s=w2406, f=w2408) -> (s? t:f=w2395:i32)
        n1563 = feedback-in #10(w2395) -> ()
        n1564 = feedback #11() -> (w2396:waveform(dbl))  [unwired: 1 out]
        n1565 = case shown="Default" w2393 {
          tunnel: [w2411 w2414] -> w2397
          tunnel: w2396 -> [w2413 _]
          tunnel: w2392 -> [w2412 w2414]
          frame Default {
            n1566 = call-poly <vilib>:"Append Waveforms.vi"("waveform B"=w2412, "waveform A"=w2413) -> ("waveform out"=w2411:waveform(dbl))  [unwired: 1 in, 8 out]
          }
          frame 1 {
          }
        }
        n1567 = feedback-in #11(w2397) -> ()
        n1568 = case shown="True" w2406 {
          tunnel: w2397 -> [_ w2410]
          frame False {
          }
          frame True {
            n1569 = call-poly <vilib>:"Mean.vi"("X"=w2410) -> ("mean"=→"Slow mean":dbl)  [unwired: 1 out]
          }
        }
      }
    }
    n1570 = case "For plotting results of scanning MCL" shown="True" w2137 {
      tunnel: w2136 -> [_ w2922]
      tunnel: w2053 -> [_ w3018]
      tunnel: w2145 -> [_ _]
      tunnel: w2014 -> [_ w2992]
      tunnel: w1989 -> [_ w2923]
      tunnel: w1988 -> [_ w2896]
      frame False {
      }
      frame True {
        w2903 = u32 0 items=["Horizontal", "Vertical", "Central", "1st Diagonal", "2nd Diagonal"] ("Type of Symmetry")
        w2931 = u32 0 items=["Horizontal", "Vertical", "Central", "1st Diagonal", "2nd Diagonal"] ("Type of Symmetry")
        w2934 = u32 0 items=["Horizontal", "Vertical", "Central", "1st Diagonal", "2nd Diagonal"] ("Type of Symmetry")
        w2963 = u32 0 items=["Horizontal", "Vertical", "Central", "1st Diagonal", "2nd Diagonal"] ("Type of Symmetry")
        n1571 = Index Array(array=w2992, index=10) -> (element=w2998:waveform(dbl))
        n1572 = Index Array(array=w2992, index=11) -> (element=w2995:waveform(dbl))
        n1573 = local read "Cycles/step (MCL)"() -> (w2948:u64)
        n1574 = Index Array(array=w2992, index="Channel") -> (element=w2994:waveform(dbl))
        n1575 = Unbundle(w2896) -> ("New Image"=w2895:T2, "New Image"=w2894:T2, "New Image"=w2893:T2, "New Image"=w2892:T2)
        n1576 = Unbundle By Name(w2998) -> ("Y"=w2950:dbl[])
        n1577 = Unbundle By Name(w2995) -> ("Y"=w2952:dbl[])
        n1578 = Unbundle By Name(w2994) -> ("Y"=w2957:dbl[])
        n1579 = call "downsample 1D array - double.vi"("Ave N"=w2948, "Array In"=w2950) -> ("Array Out"=w2949:dbl[])  [unwired: 1 out]
        n1580 = call "downsample 1D array - double.vi"("Ave N"=w2948, "Array In"=w2952) -> ("Array Out"=w2951:dbl[])  [unwired: 1 out]
        n1581 = call "downsample 1D array - double.vi"("Ave N"=w2948, "Array In"=w2957) -> ("Array Out"=w2956:dbl[])  [unwired: 1 out]
        n1582 = feedback #12(w3018) -> (w3019:dbl[])
        n1583 = Build Array (concatenate)(w3019, w3018) -> (w3000:dbl[])
        n1584 = feedback #13(w2923) -> (w2925:dbl[])
        n1585 = Build Array (concatenate)(w2925, w2923) -> (w2924:dbl[])
        n1586 = local read "Scan steps (MCL)"() -> (w2905:u64)
        n1587 = Select(t=w3018, s=w2922, f=w3000) -> (s? t:f=w3004:dbl[])
        n1588 = feedback-in #12(w3004) -> ()
        n1589 = Select(t=w2923, s=w2922, f=w2924) -> (s? t:f=w2906:dbl[])
        n1590 = feedback-in #13(w2906) -> ()
        n1591 = local read "Scan lines (y)"() -> (w2891:u64)
        n1592 = local read "N APD Samp/step"() -> (w2907:dbl)
        n1593 = feedback #14(w2949) -> (w3006:dbl[])
        n1594 = Build Array (concatenate)(w3006, w2949) -> (w2997:dbl[])
        n1595 = feedback #15(w2956) -> (w3016:dbl[])
        n1596 = Build Array (concatenate)(w3016, w2956) -> (w3015:dbl[])
        n1597 = feedback #16(w2951) -> (w3008:dbl[])
        n1598 = Build Array (concatenate)(w3008, w2951) -> (w3009:dbl[])
        n1599 = Select(t=w2949, s=w2922, f=w2997) -> (s? t:f=w2953:dbl[])
        n1600 = feedback-in #14(w2953) -> ()
        n1601 = Select(t=w2956, s=w2922, f=w3015) -> (s? t:f=w2955:dbl[])
        n1602 = feedback-in #15(w2955) -> ()
        n1603 = Select(t=w2951, s=w2922, f=w3009) -> (s? t:f=w2954:dbl[])
        n1604 = feedback-in #16(w2954) -> ()
        n1605 = Multiply(x=w2905, y=u64 2) -> (x*y=w2890:u64)
        n1606 = call "integrate 1D array interval - double.vi"("Ave N"=w2907, "Array In"=w2906) -> ("Array Out"=w2918:dbl[])  [unwired: 1 out]
        n1607 = call "integrate 1D array interval - double.vi"("Ave N"=w2907, "Array In"=w3004) -> ("Array Out"=w3003:dbl[])  [unwired: 1 out]
        n1608 = Array Size(array=w2918) -> (size(s)=w2919:i32)
        n1609 = Array Size(array=w3003) -> (size(s)=w3005:i32)
        n1610 = Multiply(x=w2891, y=w2890) -> (x*y=w2921:u64)
        n1611 = Multiply(x=w2891, y=w2890) -> (x*y=w3013:u64)
        n1612 = call-poly <vilib>:"Mean.vi"("X"=w2953) -> ("mean"=w2937:dbl)  [unwired: 1 out]
        n1613 = Subtract(x=w2921, y=w2919) -> (x-y=w2912:u64)
        n1614 = call-poly <vilib>:"Mean.vi"("X"=w2955) -> ("mean"=w2942:dbl)  [unwired: 1 out]
        n1615 = call-poly <vilib>:"Mean.vi"("X"=w2954) -> ("mean"=w2940:dbl)  [unwired: 1 out]
        n1616 = call-poly <vilib>:"Mean.vi"("X"=w2918) -> ("mean"=w2909:dbl)  [unwired: 1 out]
        n1617 = Subtract(x=w3013, y=w3005) -> (x-y=w2947:u64)
        n1618 = call-poly <vilib>:"Mean.vi"("X"=w3003) -> ("mean"=w2944:dbl)  [unwired: 1 out]
        n1619 = Initialize Array(1.0 ("element"), w2912) -> (w2908:dbl[])
        n1620 = Initialize Array(1.0 ("element"), w2947) -> (w2938:dbl[])
        n1621 = Multiply(x=w2908, y=w2909) -> (x*y=w2910:dbl[])
        n1622 = Multiply(x=w2938, y=w2940) -> (x*y=w2941:dbl[])
        n1623 = Multiply(x=w2938, y=w2942) -> (x*y=w2943:dbl[])
        n1624 = Multiply(x=w2938, y=w2937) -> (x*y=w2939:dbl[])
        n1625 = Multiply(x=w2938, y=w2944) -> (x*y=w2945:dbl[])
        n1626 = Build Array (concatenate)(w2953, w2939) -> (w3007:dbl[])
        n1627 = Build Array (concatenate)(w2955, w2943) -> (w3011:dbl[])
        n1628 = Build Array (concatenate)(w2954, w2941) -> (w3010:dbl[])
        n1629 = Build Array (concatenate)(w2918, w2910) -> (w2920:dbl[])
        n1630 = Build Array (concatenate)(w3003, w2945) -> (w3012:dbl[])
        n1631 = Reshape Array(w3007, w2891, w2890) -> (w2973:dbl[][])
        n1632 = Reshape Array(w2920, w2891, w2890) -> (w2916:dbl[][])
        n1633 = Reshape Array(w3011, w2891, w2890) -> (w2965:dbl[][])
        n1634 = Reshape Array(w3010, w2891, w2890) -> (w2980:dbl[][])
        n1635 = Reshape Array(w3012, w2891, w2890) -> (w2990:dbl[][])
        n1636 = Array Subset(array=w2980, index (col)=0 ("index"), length (col)=w2905) -> (w2985:dbl[][])  [unwired: 2 in]
        n1637 = Array Subset(array=w2980, index (col)=w2905) -> (w2983:dbl[][])  [unwired: 3 in]
        n1638 = Array Subset(array=w2965, index (col)=0 ("index"), length (col)=w2905) -> (w2971:dbl[][])  [unwired: 2 in]
        n1639 = Array Subset(array=w2965, index (col)=w2905) -> (w2969:dbl[][])  [unwired: 3 in]
        n1640 = Array Subset(array=w2916, index (col)=0 ("index"), length (col)=w2905) -> (w2915:dbl[][])  [unwired: 2 in]
        n1641 = Array Subset(array=w2916, index (col)=w2905) -> (w2913:dbl[][])  [unwired: 3 in]
        n1642 = Array Subset(array=w2990, index (col)=0 ("index"), length (col)=w2905) -> (w2989:dbl[][])  [unwired: 2 in]
        n1643 = Array Subset(array=w2990, index (col)=w2905) -> (w2987:dbl[][])  [unwired: 3 in]
        n1644 = Array Subset(array=w2973, index (col)=0 ("index"), length (col)=w2905) -> (w2978:dbl[][])  [unwired: 2 in]
        n1645 = Array Subset(array=w2973, index (col)=w2905) -> (w2976:dbl[][])  [unwired: 3 in]
        n1646 = for {
          tunnel: w2985 -> [w3027] mode=indexing
          tunnel: [w3026] -> w2984 mode=indexing
          workers-P: _ -> [_]
          n1647 = Reverse 1D Array(array=w3027) -> (reversed array=w3026:dbl[])
        }
        n1648 = for {
          tunnel: w2971 -> [w3023] mode=indexing
          tunnel: [w3022] -> w2970 mode=indexing
          workers-P: _ -> [_]
          n1649 = Reverse 1D Array(array=w3023) -> (reversed array=w3022:dbl[])
        }
        n1650 = for {
          tunnel: w2915 -> [w3021] mode=indexing
